vi "Main_v2_AE.vi"() -> ()   [LabVIEW 2023]
uses:
  AD2_MSO_SDK_class/MSOConfig.ctl
  AD2_MSO_SDK_class/AD2TriggerSources.ctl
  AD2_MSO_SDK_class/MSORangeCh.ctl
  AD2_DO_SDK_class/DOConfigureCustomData.ctl
  AD2_DO_SDK_class/DOTrigger.ctl
  AD2_WFG_SDK_class/AD2TriggerSources.ctl
  AD2_DO_SDK_class/DOCustomData.ctl
  Application_class/Application.lvclass
  <vilib>/Utility/error.llb/Error Cluster From Error Code.vi
  <vilib>/ErrorRing/Error Ring.xnode
  AD2_SDK_class/AD2_SDK.lvclass
  TC0608_class/TC0608.lvclass
  CetoniPump_class/CetoniPump.lvclass
  AFG3022B_class/AFG3022B.lvclass
  TBS2000Series_class/TBS2000Series.lvclass
  SaveData_class/SaveData.lvclass
  AD2_DO_SDK_class/AD2_DO_SDK.lvclass
  AD2_MSO_SDK_class/AD2_MSO_SDK.lvclass
panel:
  out "Pump Status":T1(array[cluster])
  in  "Tab Control":T2(tab)=enum."Log"
  out "Peltier is On":bool
  out "Oscilloscope is On":bool
  out "Analog Discovery (Camera Trigger) is On":bool
  out "Pump is On":bool
  out "Func is On":bool
  in  "Peltier Controller":bool
  in  "Oscilloscope":bool
  in  "Function Generator":bool
  in  "Cetoni Pump":bool
  in  "Analog Discovery":bool
  in  "Initialize Instruments":bool
  in  "Function Generator":refnum<visa-resource-name>
  in  "Oscilloscope":refnum<visa-resource-name>
  in  "Peltier VISA resource name":refnum<visa-resource-name>
  in  "Device Configuration Folder":string="C:\\Users\\Public\\Documents\\QmixElements\\Projects\\default_project\\Configurations\\sinle"
  in  "Oscilloscope Test":cluster{"Source Main":i32, "Source Probe":i32}={"Source Main"=2, "Source Probe"=1} {"Source Probe" items=["Math", "Channel 1", "Channel 2", "Channel 3", "Channel 4"]; "Source Main" items=["Math", "Channel 1", "Channel 2", "Channel 3", "Channel 4"]}
  in  "ReadOscilloscopeChannel":bool
  out "Temperature (C)":dbl
  in  "Read Peltier":bool
  in  "Frequency (1000 Hz)":dbl=1000.0
  in  "Set Frequency":bool
  in  "Voltage (1 Vpp)":dbl=1.0
  in  "Set Voltage":bool
  in  "Image  Aquisition":T3={"Minimum Time between frames(s)"=10.0, "Number of Frames"=0} {"Minimum Time between frames(s)" min=0.005}
  in  "Take Images":bool
  in  "Pump: GoToLevel":bool
  in  "GoToLevelSettings":T4
  in  "index":i32
  in  "refill below level":dbl
  in  "Timeout Refill":dbl=20.0 caption="Time Target (s)"
  in  "Pump: CheckLevel&Refill":bool
  in  "Pump: Reference Move":bool
  in  "Pump: Refill":bool
  in  "Index":i32
  in  "Pump: Empty":bool
  in  "Pump: Read Status":bool
  in  "SyringeSettings":T5={"Maximum Piston Stroke (mm)"=100.0, "Inner Diameter (mm)"=12.0}
  in  "index configure syringe":i32
  in  "Pump: Configure":bool
  in  "Pump: STOP":bool
  in  "Source (1: Channel 1)":i32(ring)=1 items=["Math", "Channel 1", "Channel 2", "Channel 3", "Channel 4"]
  out "Peak-to-Peak":dbl format="%.2p"
  out "Frequency":dbl format="%.2p"
  in  "MeasurePowerOsc":bool
  out "Oscilloscope Results Test":T6 {"Probe Current" format="%.2p"; "Phase Angle" format="%.2p"; "Main Freq" format="%.2p"; "Main Volt" format="%.2p"}
  in  "Oscilloscope":T7={"Source Main"=2, "Source Probe"=1, "Source Prefocus"=2} {"Source Prefocus" items=["Math", "Channel 1", "Channel 2", "Channel 3", "Channel 4"]; "Source Probe" items=["Math", "Channel 1", "Channel 2", "Channel 3", "Channel 4"]; "Source Main" items=["Math", "Channel 1", "Channel 2", "Channel 3", "Channel 4"]}
  in  "Start Experiment":bool
  out "Temperatur (C)":dbl
  in  "Experiment Settings":T8={"Frequencies (MHz)"=[], "Camera Settings"={"Minimum Time between\n frames(s)"=10.0, "Number of Frames"=0}, "Flowrates (ul/min)"=[], "Voltages (V)"=[]} {"Camera Settings"."Minimum Time between\n frames(s)" min=0.005}
  in  "SaveFolder":path
  out "Oscilloscope Results":T9 {"Probe Current" format="%.2p"; "Phase Angle" format="%.2p"; "Main Freq" format="%.2p"; "Main Volt" format="%.2p"; "Prefocus Freq" format="%.2p"; "Prefocus Volt" format="%.2p"}
  out "LOG":string
  in  "Change Frequencies and Measure":bool
  in  "FreqAndOscilloscopeTest":T10
  in  "Oscilloscope Source":i32(ring)=1 items=["Math", "Channel 1", "Channel 2", "Channel 3", "Channel 4"]
  out "Frequency (Osc.)":dbl format="%.2p"
  out "Voltage (Osc.)":dbl format="%.2p"
  out "Voltages":dbl
  out "Frequencies":dbl
  out "temperature (C)":dbl
  in  "Time To wait":dbl
  in  "Wait":bool
  in  "Configure MSO":bool
  in  "MSO":T11={"Timing"={"Enable"=TRUE, "Samples In"=100000.0, "Sample Rate"=1250000.0, "Mode"=enum."Single Sample"}, "Trigger"={"Hysteresis"=0.0, "Trigger Level"=0.0, "Trigger Condition"=0, "Trigger Type"=0, "Trigger Channel"=0, "secTimeout"=1.0, "TrigrSrc"=enum."trigrsrcNone"}, "Range Ch1"={"idxChannel"=0, "voltOffset"=0.0, "VoltsRange"=50}, "Range Ch 2"={"idxChannel"=1, "voltOffset"=0.0, "VoltsRange"=50}} {"Range Ch 2"."VoltsRange" items=["High 50V"=50, "Low5V"=5]; "Range Ch1"."VoltsRange" items=["High 50V"=50, "Low5V"=5]; "Trigger"."Trigger Channel" items=["Channel 1"=0, "Channel 2"=1, "Both"=-1]; "Trigger"."Trigger Type" items=["Edge", "Pulse", "Transition"]; "Trigger"."Trigger Condition" items=["Rising", "Falling"]}
  in  "Read MSO":bool
  out "Waveform Graph":waveform(dbl)[](graph)
  in  "Trigg AD2":bool
  in  "Configure DO":bool
  in  "?":T14={"DO Trigger"={"secRun(0=Cont)"=0.0, "secWait"=0.0, "cRepeat(0=inf)"=0, "Repeat Trigger"=TRUE, "TrigrSrc"=enum."trigsrcPC"}, "CustomData"=[{"Data"=[FALSE, TRUE, FALSE, FALSE, FALSE, FALSE, FALSE, FALSE, FALSE, FALSE, FALSE, FALSE, FALSE, FALSE, FALSE, FALSE, FALSE, FALSE, FALSE, FALSE, FALSE, FALSE], "Freq"=1000.0, "#Bits"=100, "Enable"=TRUE, "IdleState"=0}, {"Data"=[], "Freq"=0.0, "#Bits"=0, "Enable"=FALSE, "IdleState"=0}, {"Data"=[], "Freq"=0.0, "#Bits"=0, "Enable"=FALSE, "IdleState"=0}, {"Data"=[], "Freq"=0.0, "#Bits"=0, "Enable"=FALSE, "IdleState"=0}, {"Data"=[], "Freq"=0.0, "#Bits"=0, "Enable"=FALSE, "IdleState"=0}, {"Data"=[], "Freq"=0.0, "#Bits"=0, "Enable"=FALSE, "IdleState"=0}, {"Data"=[], "Freq"=0.0, "#Bits"=0, "Enable"=FALSE, "IdleState"=0}, {"Data"=[], "Freq"=0.0, "#Bits"=0, "Enable"=FALSE, "IdleState"=0}, {"Data"=[], "Freq"=0.0, "#Bits"=0, "Enable"=FALSE, "IdleState"=0}, {"Data"=[], "Freq"=0.0, "#Bits"=0, "Enable"=FALSE, "IdleState"=0}, {"Data"=[], "Freq"=0.0, "#Bits"=0, "Enable"=FALSE, "IdleState"=0}, {"Data"=[], "Freq"=0.0, "#Bits"=0, "Enable"=FALSE, "IdleState"=0}, {"Data"=[], "Freq"=0.0, "#Bits"=0, "Enable"=FALSE, "IdleState"=0}, {"Data"=[FALSE, FALSE, FALSE, FALSE, FALSE, FALSE, FALSE, FALSE, FALSE, FALSE, FALSE, FALSE, FALSE, FALSE, FALSE, FALSE, FALSE, FALSE, FALSE, FALSE, FALSE, FALSE, FALSE], "Freq"=0.0, "#Bits"=0, "Enable"=FALSE, "IdleState"=0}, {"Data"=[FALSE, FALSE, FALSE, FALSE, FALSE, FALSE, FALSE, FALSE, FALSE, FALSE, FALSE, FALSE, FALSE, FALSE, FALSE, FALSE, FALSE, FALSE, FALSE, FALSE, FALSE, FALSE, FALSE], "Freq"=0.0, "#Bits"=0, "Enable"=FALSE, "IdleState"=0}]}
  in  "ABORT":bool
  out "Status":string="Program Started\nPlease connect to instruments"
  out "error out":errorcluster
  in  "Exit":bool
  # "Notes: \nChange frequency input to MHz\ninvestigate index in GoToLevelSettings, might be unneccesary"
  # "Instruments"
  # "Peltier"
  # "Camera"
  # "Pump"
  # "Function Generator"
  # "Oscilloscope"
  # "Not sure if this is needed if we read the oscilloscope manually instead"
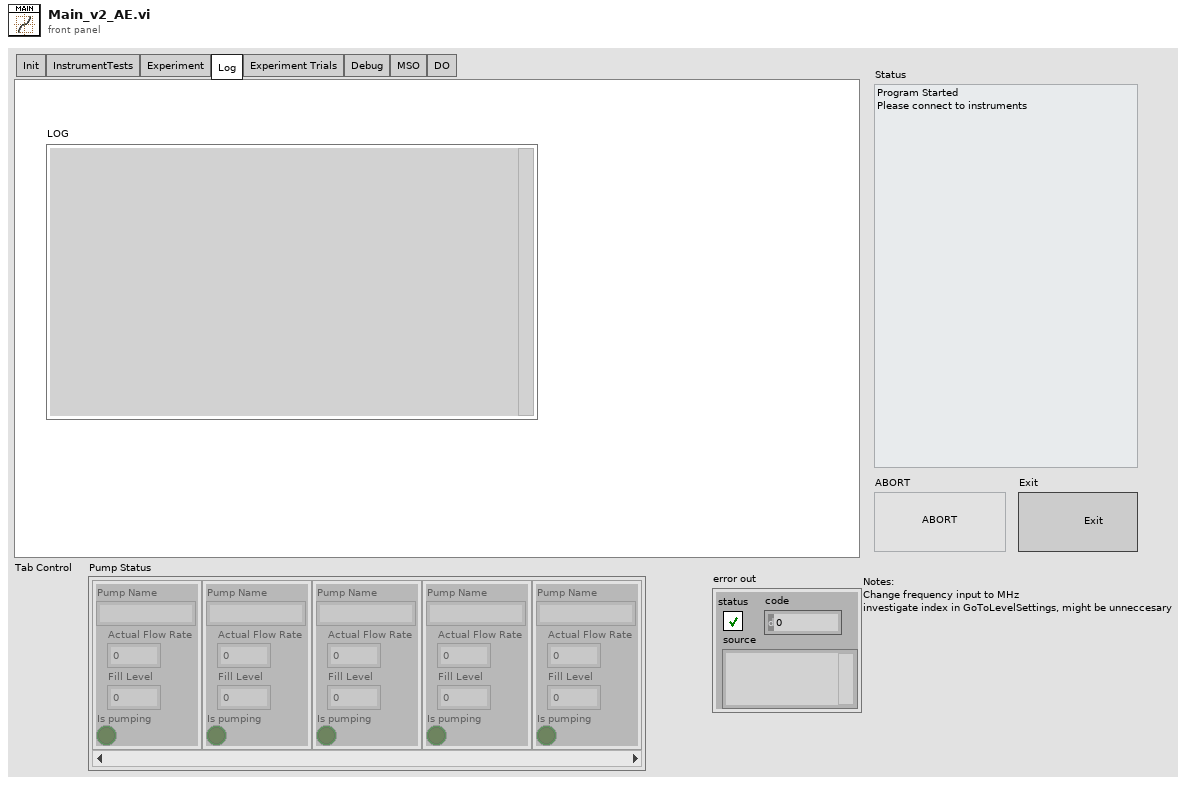
[diagram p1: front panel]
types:
  T1 = cluster{"Pump Name":string, "Actual Flow Rate":dbl, "Fill Level":dbl, "Is pumping":bool}[]
  T2 = enum32{"Init", "InstrumentTests", "Experiment", "Log", "Experiment Trials", "Debug", "MSO", "DO"}
  T3 = cluster{"Minimum Time between frames(s)":dbl, "Number of Frames":i32}
  T4 = cluster{"index":i32, "Level(ml)":dbl, "Flow":dbl}
  T5 = cluster{"Maximum Piston Stroke (mm)":dbl, "Inner Diameter (mm)":dbl}
  T6 = cluster{"Main Volt":dbl, "Main Freq":dbl, "Phase Angle":dbl, "Probe Current":dbl, "Power (Watt)":dbl}
  T7 = cluster{"Source Main":i32, "Source Probe":i32, "Source Prefocus":i32}
  T8 = cluster{"Frequencies (MHz)":dbl[], "Camera Settings":cluster{"Minimum Time between\n frames(s)":dbl, "Number of Frames":i32}, "Flowrates (ul/min)":dbl[], "Voltages (V)":dbl[]}
  T9 = cluster{"Prefocus":cluster{"Initial X":dbl, "X Increment":dbl, "Waveform Array":dbl[]}, "Prefocus Volt":dbl, "Prefocus Freq":dbl, "Main":cluster{"Initial X":dbl, "X Increment":dbl, "Waveform Array":dbl[]}, "Main Volt":dbl, "Main Freq":dbl, "Phase Angle":dbl, "Probe Current":dbl, "Power (Watt)":dbl}
  T10 = cluster{"Frequencies (MHz)":dbl[], "Voltages (V)":dbl[]}
  T11 = typedef "AD2_MSO_SDK.lvclass/MSOConfig.ctl" = cluster{"Timing":cluster{"Enable":bool, "Samples In":dbl, "Sample Rate":dbl, "Mode":enum16{"Single Sample", "Scanshift", "Multiple Samples", "Scan Screen"}}, "Trigger":cluster{"Hysteresis":dbl, "Trigger Level":dbl, "Trigger Condition":i32, "Trigger Type":i32, "Trigger Channel":i32, "secTimeout":dbl, "TrigrSrc":T12}, "Range Ch1":T13, "Range Ch 2":T13}
  T12 = typedef "AD2_MSO_SDK.lvclass/AD2TriggerSources.ctl" = enum8{"trigrsrcNone", "trigsrcPC", "trigsrcDetectorAnalogIn", "trigsrcDetectorDigitalIn", "trigsrcAnalogIn", "trigsrcDigitalIn", "trigsrcDigitalOut", "trigsrcAnalogOut1", "trigsrcAnalogOut2", "trigsrcAnalogOut3", "trigsrcAnalogOut4", "trigsrcExternal1", "trigsrcExternal2", "trigsrcExternal3", "trigsrcExternal4", ""}
  T13 = typedef "AD2_MSO_SDK.lvclass/MSORangeCh.ctl" = cluster{"idxChannel":i32, "voltOffset":dbl, "VoltsRange":u16}
  T14 = typedef "DOConfigureCustomData.ctl" = cluster{"DO Trigger":T15, "CustomData":T17}
  T15 = typedef "AD2_DO_SDK.lvclass/DOTrigger.ctl" = cluster{"secRun(0=Cont)":dbl, "secWait":dbl, "cRepeat(0=inf)":i32, "Repeat Trigger":bool, "TrigrSrc":T16}
  T16 = typedef "AD2_SDK.lvclass/AD2TriggerSources.ctl" = enum8{"trigrsrcNone", "trigsrcPC", "trigsrcDetectorAnalogIn", "trigsrcDetectorDigitalIn", "trigsrcAnalogIn", "trigsrcDigitalIn", "trigsrcDigitalOut", "trigsrcAnalogOut1", "trigsrcAnalogOut2", "trigsrcAnalogOut3", "trigsrcAnalogOut4", "trigsrcExternal1", "trigsrcExternal2", "trigsrcExternal3", "trigsrcExternal4", ""}
  T17 = typedef "AD2_DO_SDK.lvclass/DOCustomData.ctl" = cluster{"Data":bool[], "Freq":dbl, "#Bits":u32, "Enable":bool, "IdleState":u16}[]
  T18 = cluster{"Voltages":dbl, "Numeric":dbl, "selected path":path}
  T19 = cluster{"Minimum Time between frames":dbl, "Number of Frames":i32}
  T20 = cluster{"Pump Handle":i64, "Pump Name":string, "Maximum Volume":dbl, "Maximum Flow Rate":dbl, "Flow Rate":dbl, "Target Level":dbl, "Valve Handle":i64, "Has Valve?":bool, "Actual valve position":i32}[]
  T21 = cluster{"Frequency":dbl, "Peak-to-Peak":dbl, "temperature (C)":dbl}
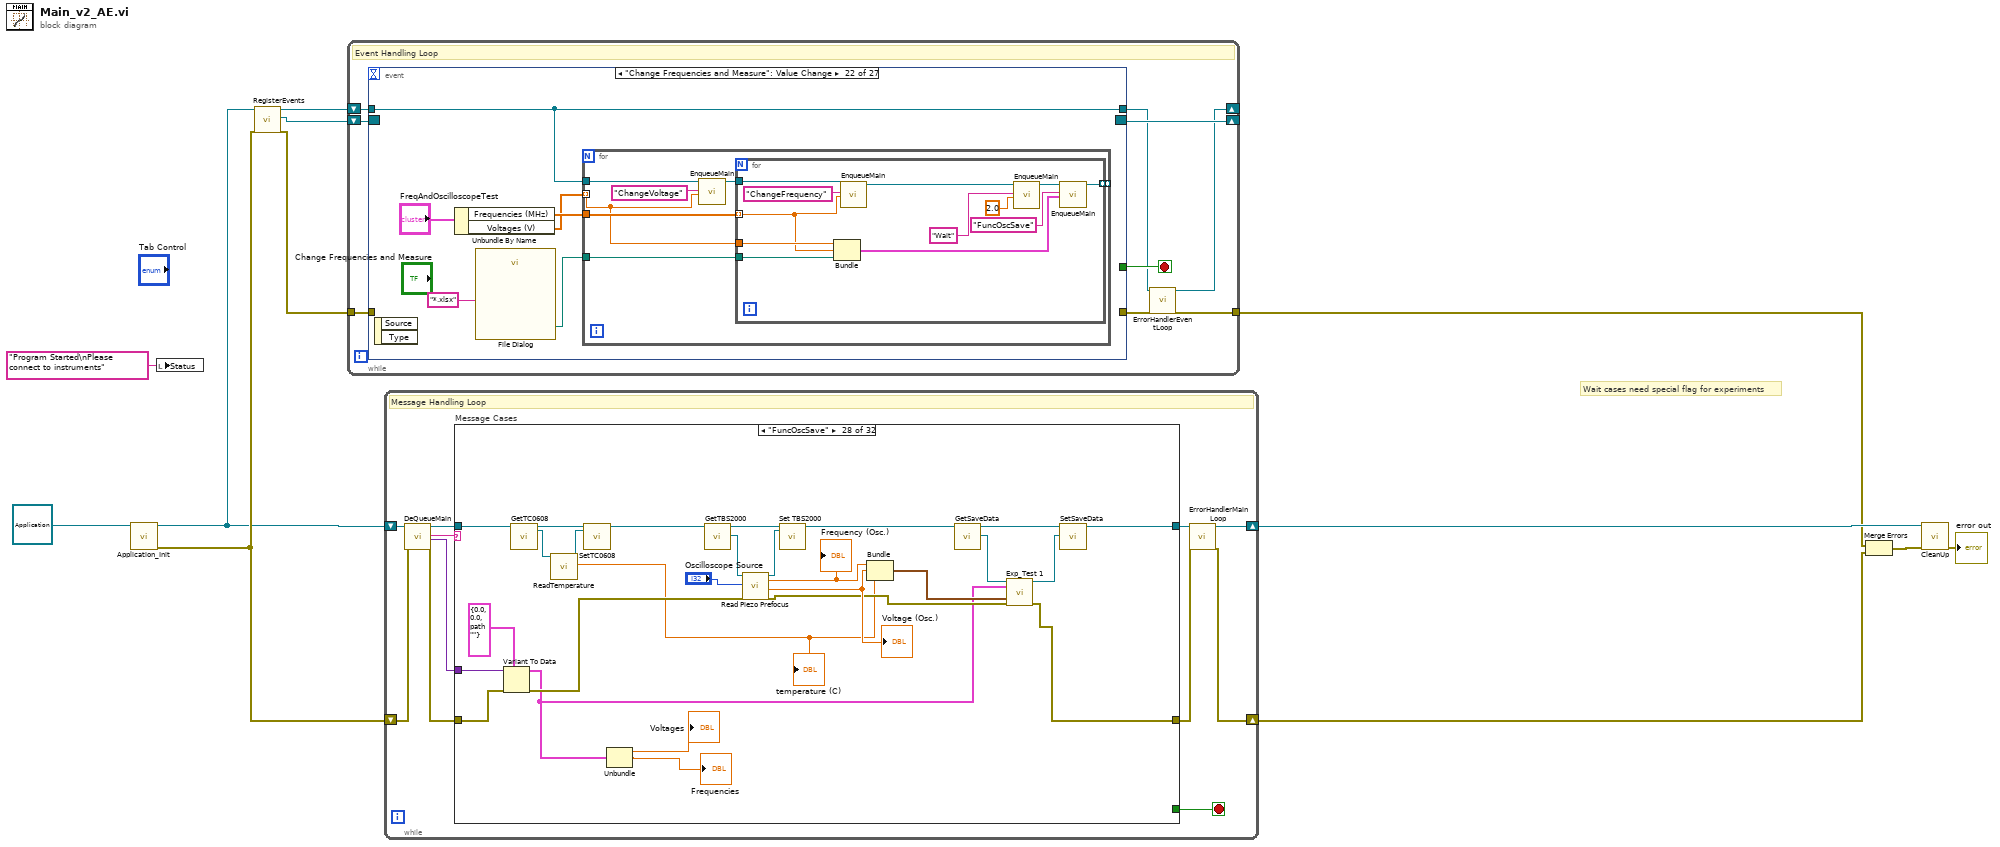
[diagram p0: block diagram]
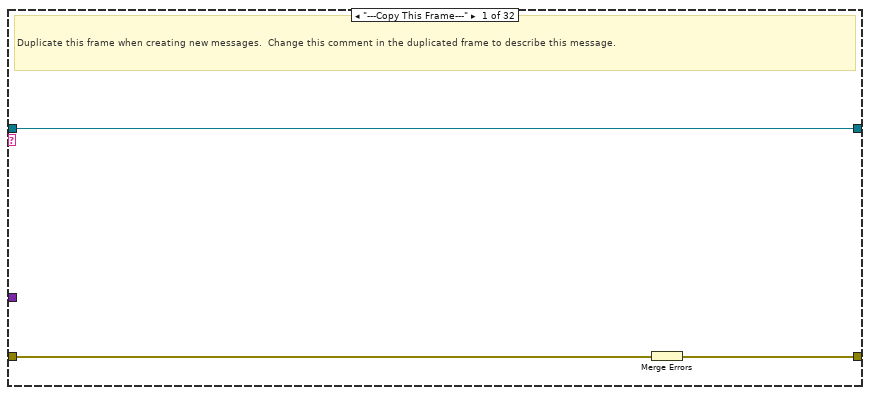
[diagram p2: hidden frame]
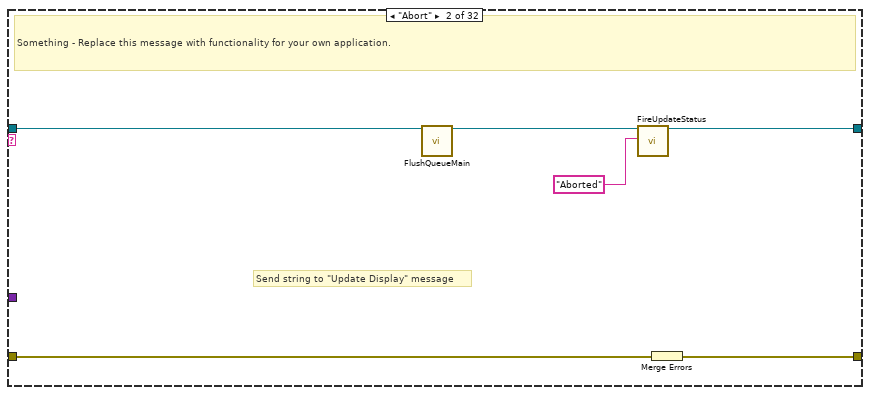
[diagram p3: hidden frame]
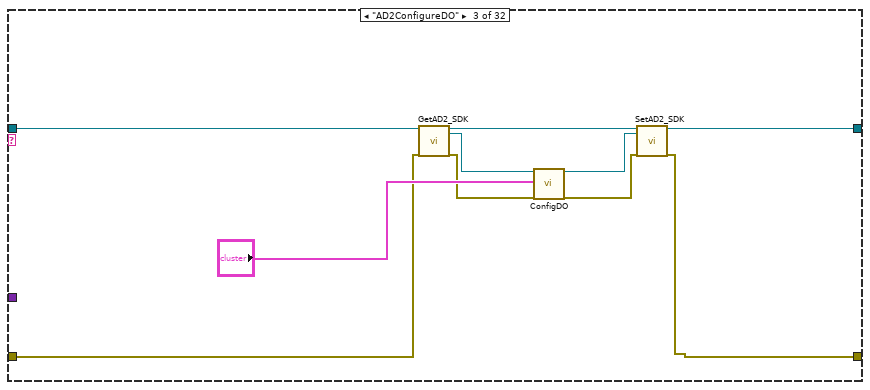
[diagram p4: hidden frame]
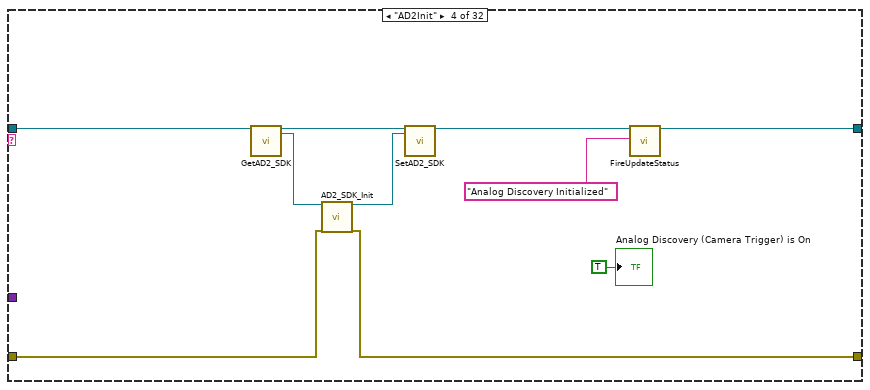
[diagram p5: hidden frame]
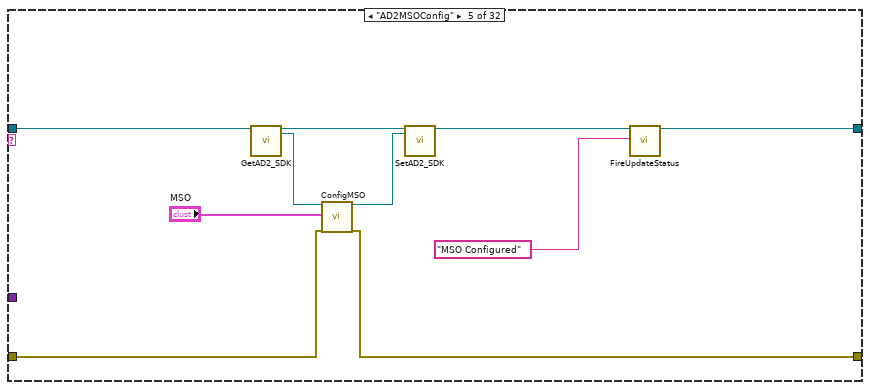
[diagram p6: hidden frame]
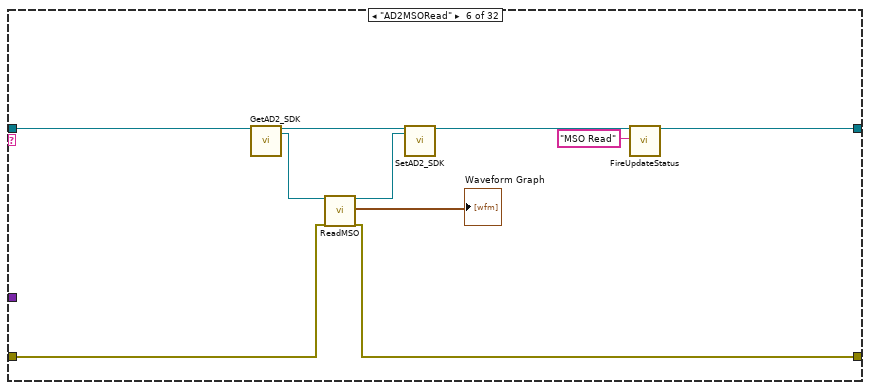
[diagram p7: hidden frame]
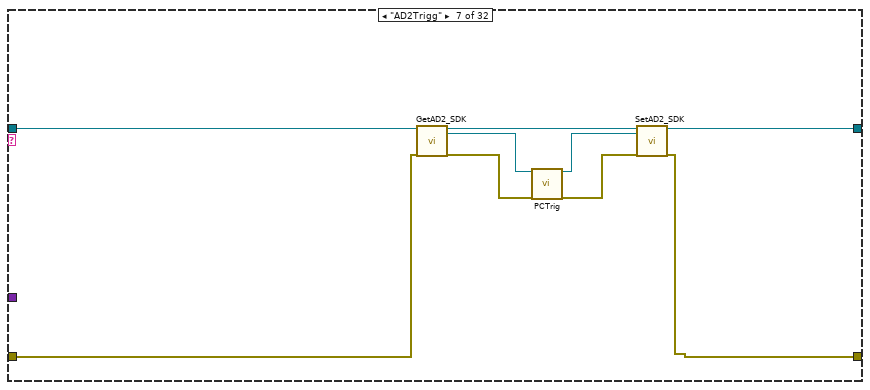
[diagram p8: hidden frame]
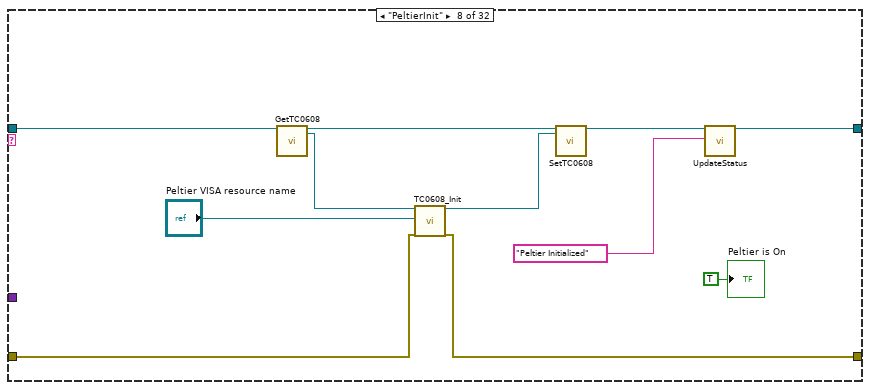
[diagram p9: hidden frame]
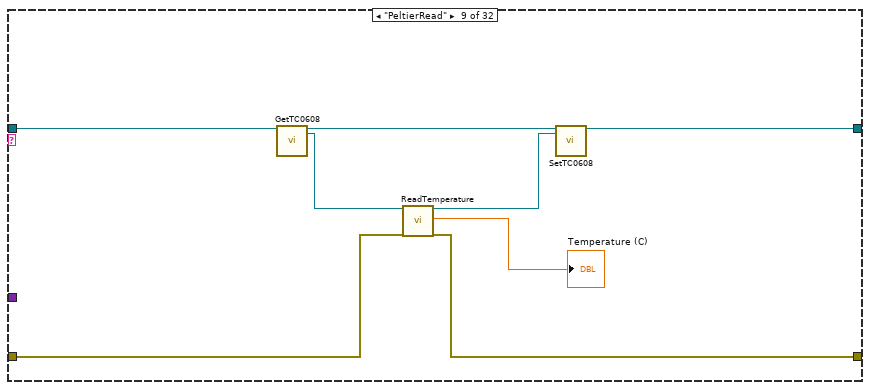
[diagram p10: hidden frame]
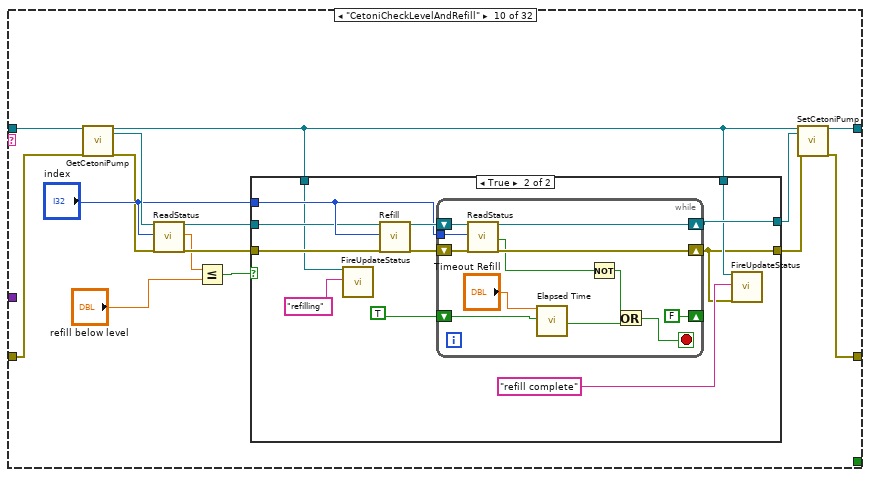
[diagram p11: hidden frame]
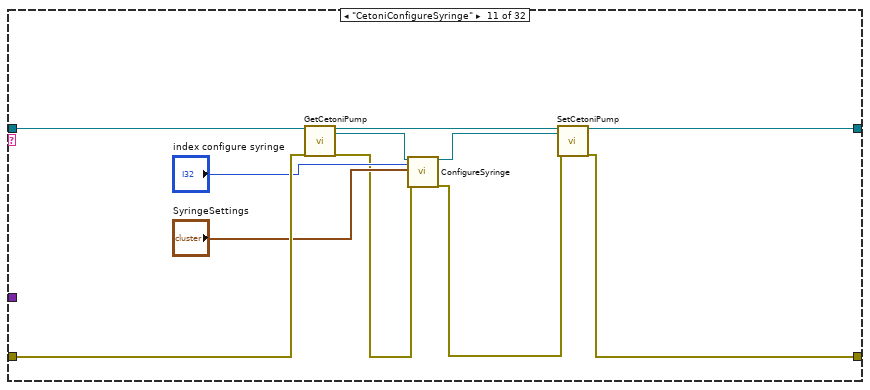
[diagram p13: hidden frame]
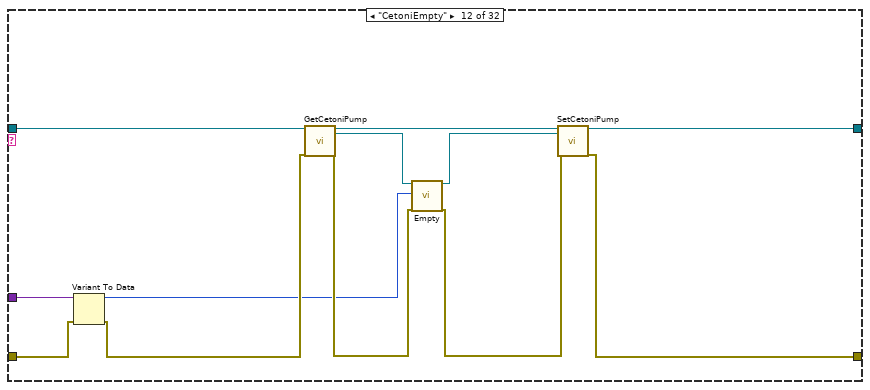
[diagram p14: hidden frame]
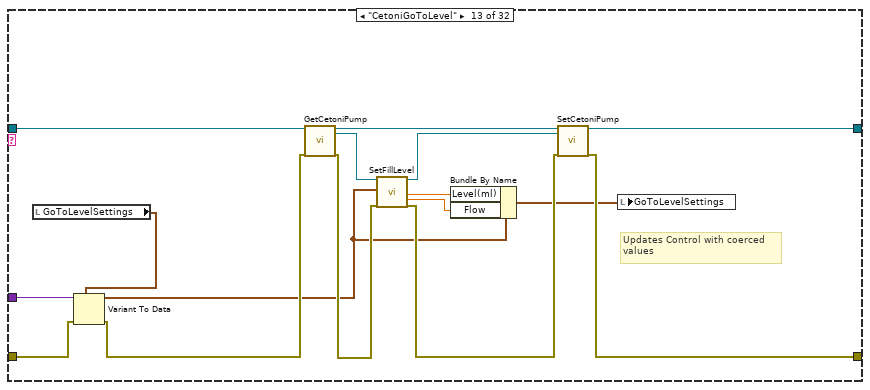
[diagram p15: hidden frame]
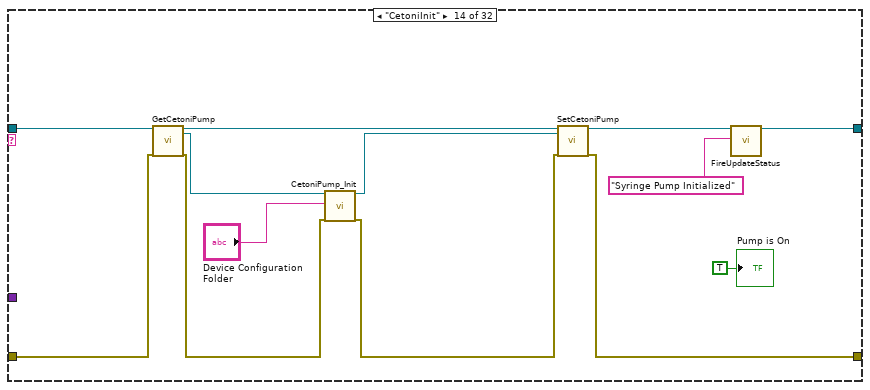
[diagram p16: hidden frame]
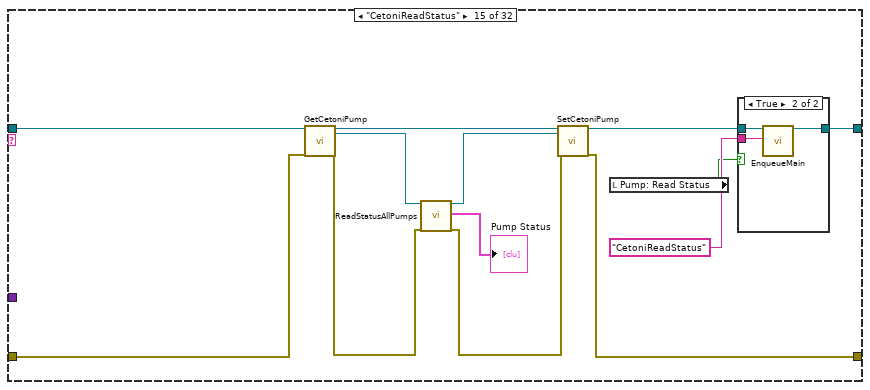
[diagram p17: hidden frame]
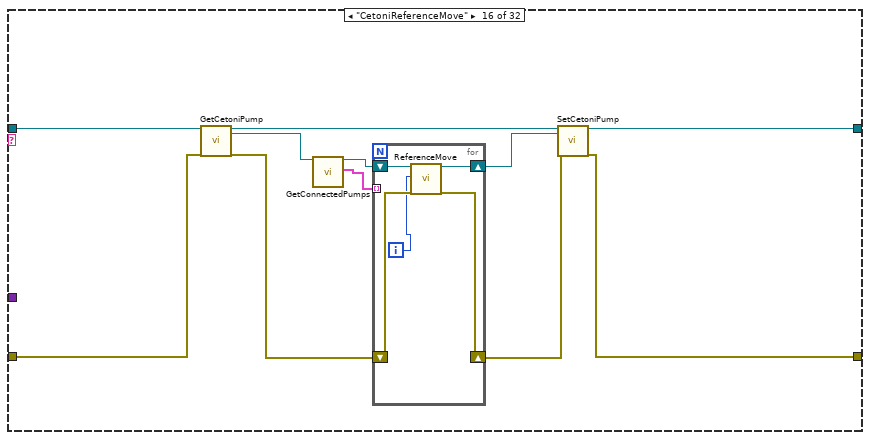
[diagram p19: hidden frame]
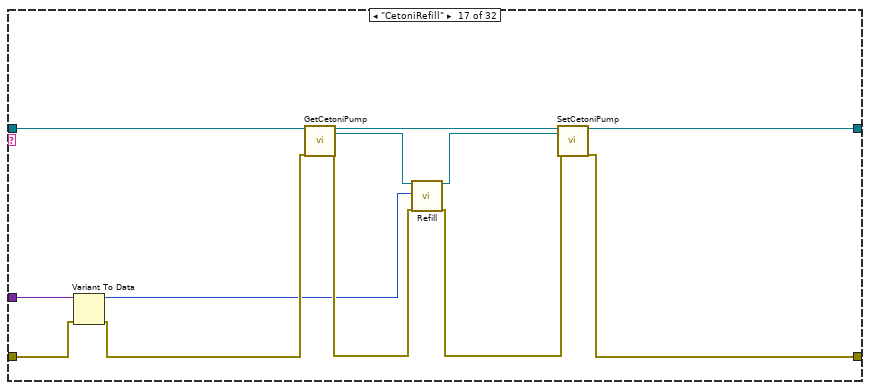
[diagram p20: hidden frame]
diagram:
  # "Wait cases need special flag for experiments"
  n1 = call "Application_Init.vi"("object in"=refnum<class "Application.lvclass"> refnum ("Application")) -> ("object out"=w2:refnum<class "Application.lvclass">, "error out"=w8:errorcluster)  [unwired: 17 in]
  n2 = local write "Status"("Program Started\nPlease connect to instruments" ("Status")) -> ()
  n3 = call-dynamic "RegisterEvents.vi"("object in"=w2, "error in (no error)"=w8) -> ("object out"=w10:refnum<class "Application.lvclass">, "Event Registration Refnum"=w11:refnum<event-registration>, "error out"=w9:errorcluster)  [unwired: 15 in]
  n4 = while {
    shift-right: [w20] -> _
    shift-left: w11 -> [w21]
    tunnel: [w15] -> w5
    shift-right: [w13] -> _
    shift-left: w10 -> [w18]
    tunnel: w9 -> [w17]
    stop <- w19 stop-if-true
    # "Event Handling Loop"
    n5 = event shown="[21] \"Change Frequencies and Measure\": Value Change" {
      selector: w21 -> [_ _ _ _ _ _ _ _ _ _ _ _ _ _ _ _ _ _ _ _ _ _ _ _ _ _ _]
      dyn-events: [_ _ _ _ _ _ _ _ _ _ _ _ _ _ _ _ _ _ _ _ _ _ _ _ _ _ _] -> w20
      timeout: _ -> [_ _ _ _ _ _ _ _ _ _ _ _ _ _ _ _ _ _ _ _ _ _ _ _ _ _ _]
      tunnel: [TRUE ("Discard?") _ _ _ _ _ _ _ _ _ _ _ _ _ _ _ _ _ _ _ _ _ _ _ _ _ _] -> w19
      tunnel: [w23 w29 w37 w42 _ _ w84 _ _ _ _ _ w104 w110 w116 w122 w127 w134 _ _ _ _ _ _ _ _ w191] -> w16
      tunnel: w18 -> [w28 w34 w36 w43 w47 w49 w88 w91 w94 w96 w98 w102 w105 w111 w117 w123 w128 w135 w146 w149 w151 w155 w180 w183 w186 w189 w194]
      tunnel: [w27 w33 w35 w43 w46 w50 w87 w91 w94 w96 w98 w101 w106 w112 w118 w124 w129 w136 w145 w148 w152 w155 w179 w182 w185 w188 w194] -> w14
      tunnel: w17 -> [w24 w30 w38 w42 _ _ w85 _ _ _ _ _ w103 w109 w115 w121 w126 w133 _ _ _ _ _ _ _ _ w192]
      event "Exit": Value Change {
        (unwired) "\"Exit\" button pressed" ("VI Stopped")
        n6 = event-data() -> ()  [unwired: 1 in, 1 out]
        n7 = call-dynamic "EnqueueMain.vi"("object in"=w28, "Message"="Exit", "error in (no error)"=w24, "Priority Message? (F)"=TRUE) -> ("object out"=w27:refnum<class "Application.lvclass">, "error out"=w23:errorcluster)  [unwired: 14 in]
      }
      event "ABORT": Value Change {
        n8 = event-data() -> ()  [unwired: 1 in, 1 out]
        n9 = call-dynamic "EnqueueMain.vi"("object in"=w34, "Message"="Abort", "error in (no error)"=w30, "Priority Message? (F)"=TRUE) -> ("object out"=w33:refnum<class "Application.lvclass">, "error out"=w29:errorcluster)  [unwired: 14 in]
      }
      event Panel Close? {
        # "Send the 'Confirm Quit' message if the user closes the panel of the VI. Discard the event so the 'Confirm Quit' message has a chance to run."
        n10 = event-data() -> ()  [unwired: 1 in, 1 out]
        n11 = call-dynamic "EnqueueMain.vi"("object in"=w36, "Message"="Confirm Quit", "error in (no error)"=w38, "Priority Message? (F)"=TRUE) -> ("object out"=w35:refnum<class "Application.lvclass">, "error out"=w37:errorcluster)  [unwired: 14 in]
        n12 = event-data("Discard?"=TRUE) -> ()  [unwired: 1 in, 1 out]
      }
      event Application Instance Close {
        # "stop the pumps if it's not automatically build into the cetoni software\nsave the log to a file"
        # "#CodeRecommended - When a project closes, all VIs within that project are aborted and leave memory. However, any code placed in this event frame is guaranteed to run to completion, so add any cleanup code that absolutely must happen here."
        n13 = event-data() -> ()  [unwired: 1 in, 1 out]
      }
      event "Wait": Value Change {
        n14 = event-data() -> ()  [unwired: 1 in, 2 out]
        n15 = call-dynamic "EnqueueMain.vi"("object in"=w47, "Message"="Wait", "Message Data"="Time To wait") -> ("object out"=w46:refnum<class "Application.lvclass">)  [unwired: 15 in, 1 out]
      }
      event "Initialize Instruments": Value Change {
        n16 = event-data() -> ()  [unwired: 1 in, 2 out]
        n17 = case shown="False" "Function Generator" {
          tunnel: w49 -> [w80 w83]
          tunnel: [w80 w82] -> w63
          tunnel: "FuncInit" ("Message") -> [_ w81]
          frame False {
          }
          frame True {
            n18 = call-dynamic "EnqueueMain.vi"("object in"=w83, "Message"=w81) -> ("object out"=w82:refnum<class "Application.lvclass">)  [unwired: 16 in, 1 out]
          }
        }
        n19 = case shown="False" "Cetoni Pump" {
          tunnel: w63 -> [w76 w79]
          tunnel: "CetoniInit" ("Message") -> [_ w78]
          tunnel: [w76 w77] -> w60
          frame False {
          }
          frame True {
            n20 = call-dynamic "EnqueueMain.vi"("object in"=w79, "Message"=w78) -> ("object out"=w77:refnum<class "Application.lvclass">)  [unwired: 16 in, 1 out]
          }
        }
        n21 = case shown="True" "Analog Discovery" {
          tunnel: w60 -> [w72 w75]
          tunnel: "AD2Init" ("Message") -> [_ w74]
          tunnel: [w72 w73] -> w56
          frame False {
          }
          frame True {
            n22 = call-dynamic "EnqueueMain.vi"("object in"=w75, "Message"=w74) -> ("object out"=w73:refnum<class "Application.lvclass">)  [unwired: 16 in, 1 out]
          }
        }
        n23 = case shown="True" "Oscilloscope" {
          tunnel: w56 -> [w68 w71]
          tunnel: "OscilloscopeInit" ("Message") -> [_ w70]
          tunnel: [w68 w69] -> w53
          frame False {
          }
          frame True {
            n24 = call-dynamic "EnqueueMain.vi"("object in"=w71, "Message"=w70) -> ("object out"=w69:refnum<class "Application.lvclass">)  [unwired: 16 in, 1 out]
          }
        }
        n25 = case shown="True" "Peltier Controller" {
          tunnel: w53 -> [w64 w67]
          tunnel: "PeltierInit" ("Message") -> [_ w66]
          tunnel: [w64 w65] -> w50
          frame False {
          }
          frame True {
            n26 = call-dynamic "EnqueueMain.vi"("object in"=w67, "Message"=w66) -> ("object out"=w65:refnum<class "Application.lvclass">)  [unwired: 16 in, 1 out]
          }
        }
      }
      event "Read Peltier": Value Change {
        n27 = event-data() -> ()  [unwired: 1 in, 2 out]
        n28 = call-dynamic "EnqueueMain.vi"("object in"=w88, "Message"="PeltierRead", "error in (no error)"=w85) -> ("object out"=w87:refnum<class "Application.lvclass">, "error out"=w84:errorcluster)  [unwired: 15 in]
      }
      event "Set Frequency": Value Change {
        n29 = event-data() -> ()  [unwired: 1 in, 2 out]
        n30 = call-dynamic "EnqueueMain.vi"("object in"=w91, "Message"="ChangeFrequency", "Message Data"="Frequency (1000 Hz)") -> ()  [unwired: 15 in, 2 out]
      }
      event "Set Voltage": Value Change {
        n31 = event-data() -> ()  [unwired: 1 in, 2 out]
        n32 = call-dynamic "EnqueueMain.vi"("object in"=w94, "Message"="ChangeVoltage", "Message Data"="Voltage (1 Vpp)") -> ()  [unwired: 15 in, 2 out]
      }
      event "MeasurePowerOsc": Value Change {
        n33 = event-data() -> ()  [unwired: 1 in, 2 out]
        n34 = call-dynamic "EnqueueMain.vi"("object in"=w96, "Message"="MeasurePowerOsc") -> ()  [unwired: 16 in, 2 out]
      }
      event "ReadOscilloscopeChannel": Value Change {
        n35 = event-data() -> ()  [unwired: 1 in, 2 out]
        n36 = call-dynamic "EnqueueMain.vi"("object in"=w98, "Message"="ReadOscilloscopeChannel") -> ()  [unwired: 16 in, 2 out]
      }
      event "Take Images": Value Change {
        n37 = event-data() -> ()  [unwired: 1 in, 2 out]
        n38 = call-dynamic "EnqueueMain.vi"("object in"=w102, "Message"="TakeNImages", "Message Data"="Image  Aquisition") -> ("object out"=w101:refnum<class "Application.lvclass">)  [unwired: 15 in, 1 out]
      }
      event "Pump: Configure": Value Change {
        n39 = event-data() -> ()  [unwired: 1 in, 2 out]
        n40 = call-dynamic "EnqueueMain.vi"("object in"=w105, "Message"="CetoniConfigureSyringe", "error in (no error)"=w103) -> ("object out"=w106:refnum<class "Application.lvclass">, "error out"=w104:errorcluster)  [unwired: 15 in]
      }
      event "Pump: GoToLevel": Value Change {
        n41 = event-data() -> ()  [unwired: 1 in, 2 out]
        n42 = call-dynamic "EnqueueMain.vi"("object in"=w111, "Message"="CetoniGoToLevel", "Message Data"="GoToLevelSettings", "error in (no error)"=w109) -> ("object out"=w112:refnum<class "Application.lvclass">, "error out"=w110:errorcluster)  [unwired: 14 in]
      }
      event "Pump: Empty": Value Change {
        n43 = event-data() -> ()  [unwired: 1 in, 2 out]
        n44 = local read "Index"() -> (w114:i32)
        n45 = call-dynamic "EnqueueMain.vi"("object in"=w117, "Message"="CetoniEmpty", "Message Data"=w114, "error in (no error)"=w115) -> ("object out"=w118:refnum<class "Application.lvclass">, "error out"=w116:errorcluster)  [unwired: 14 in]
      }
      event "Pump: Refill": Value Change {
        n46 = event-data() -> ()  [unwired: 1 in, 2 out]
        n47 = call-dynamic "EnqueueMain.vi"("object in"=w123, "Message"="CetoniRefill", "Message Data"="Index", "error in (no error)"=w121) -> ("object out"=w124:refnum<class "Application.lvclass">, "error out"=w122:errorcluster)  [unwired: 14 in]
      }
      event "Pump: Read Status": Value Change {
        n48 = event-data() -> ()  [unwired: 1 in, 2 out]
        n49 = call-dynamic "EnqueueMain.vi"("object in"=w128, "Message"="CetoniReadStatus", "error in (no error)"=w126) -> ("object out"=w129:refnum<class "Application.lvclass">, "error out"=w127:errorcluster)  [unwired: 15 in]
      }
      event "Pump: Reference Move": Value Change {
        n50 = event-data() -> ()  [unwired: 1 in, 2 out]
        n51 = Two Button Dialog(message="The pumps will perform a reference move. Please remove all syringes!!!!! ") -> (T button?=w132:bool)  [unwired: 2 in]
        n52 = case shown="True" w132 {
          tunnel: [w137 w142] -> w136
          tunnel: w135 -> [w137 w141]
          tunnel: [w138 w140] -> w134
          tunnel: w133 -> [w138 w139]
          frame False {
          }
          frame True {
            n53 = call-dynamic "EnqueueMain.vi"("object in"=w141, "Message"="CetoniReferenceMove", "error in (no error)"=w139) -> ("object out"=w142:refnum<class "Application.lvclass">, "error out"=w140:errorcluster)  [unwired: 15 in]
          }
        }
      }
      event "Pump: CheckLevel&Refill": Value Change {
        n54 = event-data() -> ()  [unwired: 1 in, 2 out]
        n55 = call-dynamic "EnqueueMain.vi"("object in"=w146, "Message"="CetoniCheckLevelAndRefill") -> ("object out"=w145:refnum<class "Application.lvclass">)  [unwired: 16 in, 1 out]
      }
      event "Pump: STOP": Value Change {
        n56 = event-data() -> ()  [unwired: 1 in, 2 out]
        n57 = call-dynamic "EnqueueMain.vi"("object in"=w149, "Message"="CetoniStopPumps") -> ("object out"=w148:refnum<class "Application.lvclass">)  [unwired: 16 in, 1 out]
      }
      event "Start Experiment": Value Change {
        # "I made a Subvi to fit screen"
        n58 = event-data() -> ()  [unwired: 1 in, 2 out]
        n59 = call-dynamic "BuildExperiment.vi"("object in"=w151, "Experiment Settings"="Experiment Settings") -> ("object out"=w152:refnum<class "Application.lvclass">)  [unwired: 16 in, 1 out]
      }
      event "Change Frequencies and Measure": Value Change {
        n60 = event-data() -> ()  [unwired: 1 in, 2 out]
        n61 = Unbundle By Name("FreqAndOscilloscopeTest") -> ("Frequencies (MHz)"=w157:dbl[], "Voltages (V)"=w156:dbl[])
        n62 = call "File Dialog"("pattern (all files)"="*.xlsx") -> ("selected path"=w153:path)  [unwired: 11 in, 3 out]
        n63 = for {
          tunnel: w157 -> [w165]
          tunnel: w156 -> [w164] mode=indexing
          tunnel: w155 -> [w163]
          tunnel: [w161] -> _ mode=indexing
          tunnel: w153 -> [w159]
          n64 = call-dynamic "EnqueueMain.vi"("object in"=w163, "Message"="ChangeVoltage", "Message Data"=w164) -> ("object out"=w162:refnum<class "Application.lvclass">)  [unwired: 15 in, 1 out]
          n65 = for {
            tunnel: w165 -> [w168] mode=indexing
            tunnel: w164 -> [w169]
            tunnel: w162 -> [w177]
            tunnel: [w176] -> w161 mode=indexing
            tunnel: w159 -> [w167]
            n66 = Bundle("Voltages"=w169, "Numeric"=w168, "selected path"=w167) -> (w166:T18)  [unwired: 1 in]
            n67 = call-dynamic "EnqueueMain.vi"("object in"=w177, "Message"="ChangeFrequency", "Message Data"=w168) -> ("object out"=w174:refnum<class "Application.lvclass">)  [unwired: 15 in, 1 out]
            n68 = call-dynamic "EnqueueMain.vi"("object in"=w174, "Message"="Wait", "Message Data"=2.0 ("Time to wait")) -> ("object out"=w173:refnum<class "Application.lvclass">)  [unwired: 15 in, 1 out]
            n69 = call-dynamic "EnqueueMain.vi"("object in"=w173, "Message"="FuncOscSave", "Message Data"=w166) -> ("object out"=w176:refnum<class "Application.lvclass">)  [unwired: 15 in, 1 out]
          }
        }
      }
      event "Configure DO": Value Change {
        n70 = event-data() -> ()  [unwired: 1 in, 2 out]
        n71 = call-dynamic "EnqueueMain.vi"("object in"=w180, "Message"="AD2ConfigureDO") -> ("object out"=w179:refnum<class "Application.lvclass">)  [unwired: 16 in, 1 out]
      }
      event "Configure MSO": Value Change {
        n72 = event-data() -> ()  [unwired: 1 in, 2 out]
        n73 = call-dynamic "EnqueueMain.vi"("object in"=w183, "Message"="AD2MSOConfig") -> ("object out"=w182:refnum<class "Application.lvclass">)  [unwired: 16 in, 1 out]
      }
      event "Read MSO": Value Change {
        n74 = event-data() -> ()  [unwired: 1 in, 2 out]
        n75 = call-dynamic "EnqueueMain.vi"("object in"=w186, "Message"="AD2MSORead") -> ("object out"=w185:refnum<class "Application.lvclass">)  [unwired: 16 in, 1 out]
      }
      event "Trigg AD2": Value Change {
        n76 = event-data() -> ()  [unwired: 1 in, 2 out]
        n77 = call-dynamic "EnqueueMain.vi"("object in"=w189, "Message"="AD2Trigg") -> ("object out"=w188:refnum<class "Application.lvclass">)  [unwired: 16 in, 1 out]
      }
      event User Event {
        n78 = event-data() -> ("Message"=w193:string, "Message Data"=w190:variant)  [unwired: 1 in]
        n79 = case shown="\"UpdateStatus\"" w193 {
          tunnel: w192 -> [w198 w207]
          tunnel: [w198 w207] -> w191
          tunnel: w190 -> [w197 _]
          frame "UpdateStatus" {
            # "I have disabled the log, it might slow down the program\nwhen it becomes to large"
            n80 = Variant To Data(type="" ("Status"), Variant=w197) -> (data=w195:string)  [unwired: 1 in, 1 out]
            "Status" <- w195
            n81 = disable-structure shown="Disabled" {
              disable-tunnel: w195 -> [w202 _]
              frame Disabled {
                n82 = Get Date/Time In Seconds() -> (seconds since 1Jan1904=w206:timestamp)
                n83 = Get Date/Time String(seconds (now)=w206) -> (time string=w203:string)  [unwired: 2 in, 1 out]
                n84 = feedback #1("" ("string")) -> (w199:string)
                n85 = Concatenate Strings(w199, "\r", w203, "\t", w202) -> (w201:string)
                "LOG" <- w201
                n86 = feedback-in #1(w201) -> ()
              }
              frame Enabled {
              }
            }
          }
          frame Default {
          }
        }
      }
    }
    n87 = call-dynamic "ErrorHandlerEventLoop.vi"("object in"=w14, "error in (no error)"=w16) -> ("object out"=w13:refnum<class "Application.lvclass">, "error out"=w15:errorcluster)  [unwired: 16 in]
  }
  n88 = while {
    shift-right: [w211] -> w7
    shift-left: w2 -> [w217]
    shift-right: [w212] -> w6
    shift-left: w8 -> [w208]
    stop <- w218 stop-if-true
    # "Message Handling Loop"
    n89 = call-dynamic "DeQueueMain.vi"("object in"=w217, "error in (no error)"=w208) -> ("object out"=w216:refnum<class "Application.lvclass">, "Message"=w215:string, "Message Data"=w214:variant, "error out"=w209:errorcluster)  [unwired: 14 in]
    n90 = case "Message Cases" shown="\"FuncOscSave\"" w215 {
      selector: w215 -> [_ _ _ _ _ _ _ _ _ _ _ _ _ _ _ _ _ _ _ _ _ _ _ _ _ _ _ _ _ _ _ w623]
      tunnel: w209 -> [w221 w226 w228 w243 w253 w262 w272 w280 w290 w307 w343 w353 w364 w387 w398 w412 w427 w438 w449 w465 w476 w478 w487 w503 w516 w519 w535 w551 w579 w587 w619 _]
      tunnel: [w220 w227 w229 w244 w254 w261 w273 w281 w289 w308 w345 w357 w373 w386 w400 w414 w431 w440 w450 w466 w471 w479 w488 w503 w515 w520 w535 w547 w568 w588 w615 w624] -> w213
      tunnel: [_ _ _ _ _ _ _ _ _ _ _ _ _ _ _ _ _ _ _ _ _ TRUE _ _ _ _ _ _ _ _ _ _] -> w218
      tunnel: w214 -> [_ _ _ _ _ _ _ _ _ _ _ w355 w366 _ _ _ w429 _ w451 w467 w475 _ _ _ _ _ _ w562 w566 w590 w621 _]
      tunnel: w216 -> [w219 w225 w237 w247 w257 w267 w276 w283 w293 w310 w347 w359 w375 w388 w401 w416 w433 w442 w452 w468 w470 w480 w492 w498 w513 w526 w532 w539 w583 w594 w617 w622]
      tunnel: [w219 w223 w235 w240 w249 w260 w274 w279 w294 w309 w346 w358 w374 w377 w390 w415 w432 w441 w447 w463 w470 w481 w484 w499 w509 w524 w533 w555 w571 w595 w612 w622] -> w210
      frame "---Copy This Frame---" {
        # "Duplicate this frame when creating new messages.  Change this comment in the duplicated frame to describe this message."
        n91 = Merge Errors(w221) -> (w220:errorcluster)
      }
      frame "Abort" {
        # "Send string to \"Update Display\" message"
        # "Something - Replace this message with functionality for your own application."
        n92 = call-dynamic "FlushQueueMain.vi"("object in"=w225) -> ("object out"=w224:refnum<class "Application.lvclass">)  [unwired: 16 in, 2 out]
        n93 = call-dynamic "FireUpdateStatus.vi"("object in"=w224, "Status"="Aborted") -> ("object out"=w223:refnum<class "Application.lvclass">)  [unwired: 16 in, 1 out]
        n94 = Merge Errors(w226) -> (w227:errorcluster)
      }
      frame "AD2ConfigureDO" {
        n95 = call-dynamic "GetAD2_SDK.vi"("object in"=w237, "error in (no error)"=w228) -> ("object out"=w236:refnum<class "Application.lvclass">, "AD2_SDK"=w233:refnum<class "AD2_SDK.lvclass">, "error out"=w232:errorcluster)  [unwired: 15 in]
        n96 = call-dynamic "ConfigDO.vi"("object in"=w233, 2:"?", "error in (no error)"=w232) -> ("object out"=w231:refnum<class "AD2_SDK.lvclass">, "error out"=w230:errorcluster)  [unwired: 15 in]
        n97 = call-dynamic "SetAD2_SDK.vi"("object in"=w236, "AD2_SDK"=w231, "error in (no error)"=w230) -> ("object out"=w235:refnum<class "Application.lvclass">, "error out"=w229:errorcluster)  [unwired: 15 in]
      }
      frame "AD2Init" {
        n98 = call-dynamic "GetAD2_SDK.vi"("object in"=w247) -> ("object out"=w246:refnum<class "Application.lvclass">, "AD2_SDK"=w242:refnum<class "AD2_SDK.lvclass">)  [unwired: 16 in, 1 out]
        n99 = call "AD2_SDK_Init.vi"("object in"=w242, "error in (no error)"=w243) -> ("object out"=w241:refnum<class "AD2_SDK.lvclass">, "error out"=w244:errorcluster)  [unwired: 16 in]
        n100 = call-dynamic "SetAD2_SDK.vi"("object in"=w246, "AD2_SDK"=w241) -> ("object out"=w245:refnum<class "Application.lvclass">)  [unwired: 16 in, 1 out]
        n101 = call-dynamic "FireUpdateStatus.vi"("object in"=w245, "Status"="Analog Discovery Initialized") -> ("object out"=w240:refnum<class "Application.lvclass">)  [unwired: 16 in, 1 out]
        "Analog Discovery (Camera Trigger) is On" <- TRUE ("Analog Discovery (Camera Trigger) is On")
      }
      frame "AD2MSOConfig" {
        n102 = call-dynamic "GetAD2_SDK.vi"("object in"=w257) -> ("object out"=w256:refnum<class "Application.lvclass">, "AD2_SDK"=w252:refnum<class "AD2_SDK.lvclass">)  [unwired: 16 in, 1 out]
        n103 = call-dynamic "ConfigMSO.vi"("object in"=w252, "variant"="MSO", "error in (no error)"=w253) -> ("object out"=w251:refnum<class "AD2_SDK.lvclass">, "error out"=w254:errorcluster)  [unwired: 15 in]
        n104 = call-dynamic "SetAD2_SDK.vi"("object in"=w256, "AD2_SDK"=w251) -> ("object out"=w255:refnum<class "Application.lvclass">)  [unwired: 16 in, 1 out]
        n105 = call-dynamic "FireUpdateStatus.vi"("object in"=w255, "Status"="MSO Configured") -> ("object out"=w249:refnum<class "Application.lvclass">)  [unwired: 16 in, 1 out]
      }
      frame "AD2MSORead" {
        n106 = call-dynamic "GetAD2_SDK.vi"("object in"=w267) -> ("object out"=w266:refnum<class "Application.lvclass">, "AD2_SDK"=w264:refnum<class "AD2_SDK.lvclass">)  [unwired: 16 in, 1 out]
        n107 = call-dynamic "ReadMSO.vi"("object in"=w264, "error in (no error)"=w262) -> ("object out"=w263:refnum<class "AD2_SDK.lvclass">, "Channels array"=→"Waveform Graph":waveform(dbl)[], "error out"=w261:errorcluster)  [unwired: 15 in]
        n108 = call-dynamic "SetAD2_SDK.vi"("object in"=w266, "AD2_SDK"=w263) -> ("object out"=w265:refnum<class "Application.lvclass">)  [unwired: 16 in, 1 out]
        n109 = call-dynamic "FireUpdateStatus.vi"("object in"=w265, "Status"="MSO Read") -> ("object out"=w260:refnum<class "Application.lvclass">)  [unwired: 16 in, 1 out]
      }
      frame "AD2Trigg" {
        n110 = call-dynamic "GetAD2_SDK.vi"("object in"=w276, "error in (no error)"=w272) -> ("object out"=w275:refnum<class "Application.lvclass">, "AD2_SDK"=w271:refnum<class "AD2_SDK.lvclass">, "error out"=w269:errorcluster)  [unwired: 15 in]
        n111 = call-dynamic "PCTrig.vi"("object in"=w271, "error in (no error)"=w269) -> ("object out"=w270:refnum<class "AD2_SDK.lvclass">, "error out"=w268:errorcluster)  [unwired: 16 in]
        n112 = call-dynamic "SetAD2_SDK.vi"("object in"=w275, "AD2_SDK"=w270, "error in (no error)"=w268) -> ("object out"=w274:refnum<class "Application.lvclass">, "error out"=w273:errorcluster)  [unwired: 15 in]
      }
      frame "PeltierInit" {
        n113 = call-dynamic "GetTC0608.vi"("object in"=w283) -> ("object out"=w285:refnum<class "Application.lvclass">, "TC0608"=w287:refnum<class "TC0608.lvclass">)  [unwired: 16 in, 1 out]
        n114 = call "TC0608_Init.vi"("object in"=w287, "VISA resource name"="Peltier VISA resource name", "error in (no error)"=w280) -> ("object out"=w286:refnum<class "TC0608.lvclass">, "error out"=w281:errorcluster)  [unwired: 15 in]
        n115 = call-dynamic "SetTC0608.vi"("object in"=w285, "TC0608"=w286) -> ("object out"=w284:refnum<class "Application.lvclass">)  [unwired: 16 in, 1 out]
        n116 = call-dynamic "UpdateStatus.vi"("object in"=w284, "Status"="Peltier Initialized") -> ("object out"=w279:refnum<class "Application.lvclass">)  [unwired: 16 in, 1 out]
        "Peltier is On" <- TRUE ("Peltier is On")
      }
      frame "PeltierRead" {
        n117 = call-dynamic "GetTC0608.vi"("object in"=w293) -> ("object out"=w295:refnum<class "Application.lvclass">, "TC0608"=w292:refnum<class "TC0608.lvclass">)  [unwired: 16 in, 1 out]
        n118 = call-dynamic "ReadTemperature.vi"("object in"=w292, "error in (no error)"=w290) -> ("object out"=w291:refnum<class "TC0608.lvclass">, "temperature (C)"=→"Temperature (C)":dbl, "error out"=w289:errorcluster)  [unwired: 15 in]
        n119 = call-dynamic "SetTC0608.vi"("object in"=w295, "TC0608"=w291) -> ("object out"=w294:refnum<class "Application.lvclass">)  [unwired: 16 in, 1 out]
      }
      frame "CetoniCheckLevelAndRefill" {
        n120 = call-dynamic "GetCetoniPump.vi"("object in"=w310, "error in (no error)"=w307) -> ("object out"=w296:refnum<class "Application.lvclass">, "CetoniPump"=w306:refnum<class "CetoniPump.lvclass">, "error out"=w298:errorcluster)  [unwired: 15 in]
        n121 = call-dynamic "ReadStatus.vi"("object in"=w306, "index"="index", "error in (no error)"=w298) -> ("object out"=w304:refnum<class "CetoniPump.lvclass">, "Fill Level"=w301:dbl, "error out"=w303:errorcluster)  [unwired: 12 in, 2 out]
        n122 = Less Or Equal?(x=w301, y="refill below level") -> (x <= y?=w302:bool)
        n123 = case shown="True" w302 {
          tunnel: "index" -> [_ w323]
          tunnel: w304 -> [w312 w319]
          tunnel: w303 -> [w311 w321]
          tunnel: [w312 w316] -> w299
          tunnel: [w311 w313] -> w297
          tunnel: w296 -> [_ w318]
          tunnel: w296 -> [_ w315]
          frame False {
          }
          frame True {
            n124 = call-dynamic "FireUpdateStatus.vi"("object in"=w318, "Status"="refilling") -> ()  [unwired: 16 in, 2 out]
            n125 = call-dynamic "Refill.vi"("object in"=w319, "index"=w323, "error in (no error)"=w321) -> ("object out"=w324:refnum<class "CetoniPump.lvclass">, "error out"=w322:errorcluster)  [unwired: 15 in]
            n126 = while {
              tunnel: w323 -> [w335]
              shift-right: [w325] -> w316
              shift-left: w324 -> [w336]
              shift-right: [w333] -> w313
              shift-left: w322 -> [w334]
              shift-right: [FALSE] -> _
              shift-left: TRUE -> [w327]
              stop <- w328 stop-if-true
              n127 = call-dynamic "ReadStatus.vi"("object in"=w336, "index"=w335, "error in (no error)"=w334) -> ("object out"=w325:refnum<class "CetoniPump.lvclass">, "Is pumping"=w331:bool, "error out"=w333:errorcluster)  [unwired: 12 in, 2 out]
              n128 = call "Elapsed Time"("Time Target (s)"="Timeout Refill", "Reset"=w327) -> ("Time has Elapsed"=w329:bool)  [unwired: 10 in, 7 out]
              n129 = Not(x=w331) -> (.not. x?=w330:bool)
              n130 = Or(x=w330, y=w329) -> (x .or. y?=w328:bool)
            }
            n131 = call-dynamic "FireUpdateStatus.vi"("object in"=w315, "Status"="refill complete", "error in (no error)"=w313) -> ()  [unwired: 15 in, 2 out]
          }
        }
        n132 = call-dynamic "SetCetoniPump.vi"("object in"=w296, "CetoniPump"=w299, "error in (no error)"=w297) -> ("object out"=w309:refnum<class "Application.lvclass">, "error out"=w308:errorcluster)  [unwired: 15 in]
      }
      frame "CetoniConfigureSyringe" {
        n133 = call-dynamic "GetCetoniPump.vi"("object in"=w347, "error in (no error)"=w343) -> ("object out"=w344:refnum<class "Application.lvclass">, "CetoniPump"=w342:refnum<class "CetoniPump.lvclass">, "error out"=w338:errorcluster)  [unwired: 15 in]
        n134 = call-dynamic "ConfigureSyringe.vi"("object in"=w342, "index"="index configure syringe", "SyringeSettings"="SyringeSettings", "error in (no error)"=w338) -> ("object out"=w341:refnum<class "CetoniPump.lvclass">, "error out"=w337:errorcluster)  [unwired: 14 in]
        n135 = call-dynamic "SetCetoniPump.vi"("object in"=w344, "CetoniPump"=w341, "error in (no error)"=w337) -> ("object out"=w346:refnum<class "Application.lvclass">, "error out"=w345:errorcluster)  [unwired: 15 in]
      }
      frame "CetoniEmpty" {
        n136 = Variant To Data(error in=w353, Variant=w355) -> (data=w348:i32, error out=w354:errorcluster)  [unwired: 1 in]
        n137 = call-dynamic "GetCetoniPump.vi"("object in"=w359, "error in (no error)"=w354) -> ("object out"=w356:refnum<class "Application.lvclass">, "CetoniPump"=w352:refnum<class "CetoniPump.lvclass">, "error out"=w350:errorcluster)  [unwired: 15 in]
        n138 = call-dynamic "Empty.vi"("object in"=w352, "index"=w348, "error in (no error)"=w350) -> ("object out"=w351:refnum<class "CetoniPump.lvclass">, "error out"=w349:errorcluster)  [unwired: 15 in]
        n139 = call-dynamic "SetCetoniPump.vi"("object in"=w356, "CetoniPump"=w351, "error in (no error)"=w349) -> ("object out"=w358:refnum<class "Application.lvclass">, "error out"=w357:errorcluster)  [unwired: 15 in]
      }
      frame "CetoniGoToLevel" {
        # "Updates Control with coerced\nvalues"
        n140 = local read "GoToLevelSettings"() -> (w363:T4)
        n141 = Variant To Data(error in=w364, type=w363, Variant=w366) -> (data=w362:T4, error out=w365:errorcluster)
        n142 = call-dynamic "GetCetoniPump.vi"("object in"=w375, "error in (no error)"=w365) -> ("object out"=w372:refnum<class "Application.lvclass">, "CetoniPump"=w369:refnum<class "CetoniPump.lvclass">, "error out"=w371:errorcluster)  [unwired: 15 in]
        n143 = call-dynamic "SetFillLevel.vi"("object in"=w369, "GoToLevelSettings"=w362, "error in (no error)"=w371) -> ("object out"=w368:refnum<class "CetoniPump.lvclass">, "Coerced Level"=w367:dbl, "Coerced Flow"=w361:dbl, "error out"=w370:errorcluster)  [unwired: 12 in, 1 out]
        n144 = Bundle By Name(cluster=w362, "Level(ml)"=w367, "Flow"=w361) -> (w360:T4)
        n145 = call-dynamic "SetCetoniPump.vi"("object in"=w372, "CetoniPump"=w368, "error in (no error)"=w370) -> ("object out"=w374:refnum<class "Application.lvclass">, "error out"=w373:errorcluster)  [unwired: 15 in]
        n146 = local write "GoToLevelSettings"(w360) -> ()
      }
      frame "CetoniInit" {
        n147 = call-dynamic "GetCetoniPump.vi"("object in"=w388, "error in (no error)"=w387) -> ("object out"=w385:refnum<class "Application.lvclass">, "CetoniPump"=w384:refnum<class "CetoniPump.lvclass">, "error out"=w382:errorcluster)  [unwired: 15 in]
        n148 = call "CetoniPump_Init.vi"("object in"=w384, "Device Configuration Path"="Device Configuration Folder", "error in (no error)"=w382) -> ("object out"=w383:refnum<class "CetoniPump.lvclass">, "error out"=w381:errorcluster)  [unwired: 15 in]
        n149 = call-dynamic "SetCetoniPump.vi"("object in"=w385, "CetoniPump"=w383, "error in (no error)"=w381) -> ("object out"=w378:refnum<class "Application.lvclass">, "error out"=w386:errorcluster)  [unwired: 15 in]
        n150 = call-dynamic "FireUpdateStatus.vi"("object in"=w378, "Status"="Syringe Pump Initialized") -> ("object out"=w377:refnum<class "Application.lvclass">)  [unwired: 16 in, 1 out]
        "Pump is On" <- TRUE ("Pump is On")
      }
      frame "CetoniReadStatus" {
        n151 = call-dynamic "GetCetoniPump.vi"("object in"=w401, "error in (no error)"=w398) -> ("object out"=w399:refnum<class "Application.lvclass">, "CetoniPump"=w397:refnum<class "CetoniPump.lvclass">, "error out"=w395:errorcluster)  [unwired: 15 in]
        n152 = call-dynamic "ReadStatusAllPumps.vi"("object in"=w397, "error in (no error)"=w395) -> ("object out"=w396:refnum<class "CetoniPump.lvclass">, "Array"=→"Pump Status":T1, "error out"=w394:errorcluster)  [unwired: 15 in]
        n153 = call-dynamic "SetCetoniPump.vi"("object in"=w399, "CetoniPump"=w396, "error in (no error)"=w394) -> ("object out"=w391:refnum<class "Application.lvclass">, "error out"=w400:errorcluster)  [unwired: 15 in]
        n154 = local read "Pump: Read Status"() -> (w389:bool)
        n155 = case shown="True" w389 {
          tunnel: "CetoniReadStatus" ("Message") -> [_ w405]
          tunnel: w391 -> [w402 w404]
          tunnel: [w402 w403] -> w390
          frame False {
          }
          frame True {
            n156 = call-dynamic "EnqueueMain.vi"("object in"=w404, "Message"=w405) -> ("object out"=w403:refnum<class "Application.lvclass">)  [unwired: 16 in, 1 out]
          }
        }
      }
      frame "CetoniReferenceMove" {
        n157 = call-dynamic "GetCetoniPump.vi"("object in"=w416, "error in (no error)"=w412) -> ("object out"=w413:refnum<class "Application.lvclass">, "CetoniPump"=w411:refnum<class "CetoniPump.lvclass">, "error out"=w408:errorcluster)  [unwired: 15 in]
        n158 = call-dynamic "GetConnectedPumps.vi"("object in"=w411) -> ("object out"=w410:refnum<class "CetoniPump.lvclass">, "ConnectedPumps"=w406:T20)  [unwired: 16 in, 1 out]
        n159 = for {
          shift-right: [w420] -> w409
          shift-left: w410 -> [w421]
          shift-right: [w418] -> w407
          shift-left: w408 -> [w419]
          tunnel: w406 -> [_] mode=indexing
          i -> [w417]
          n160 = call-dynamic "ReferenceMove.vi"("object in"=w421, "index"=w417, "error in (no error)"=w419) -> ("object out"=w420:refnum<class "CetoniPump.lvclass">, "error out"=w418:errorcluster)  [unwired: 15 in]
        }
        n161 = call-dynamic "SetCetoniPump.vi"("object in"=w413, "CetoniPump"=w409, "error in (no error)"=w407) -> ("object out"=w415:refnum<class "Application.lvclass">, "error out"=w414:errorcluster)  [unwired: 15 in]
      }
      frame "CetoniRefill" {
        n162 = Variant To Data(error in=w427, Variant=w429) -> (data=w422:i32, error out=w428:errorcluster)  [unwired: 1 in]
        n163 = call-dynamic "GetCetoniPump.vi"("object in"=w433, "error in (no error)"=w428) -> ("object out"=w430:refnum<class "Application.lvclass">, "CetoniPump"=w426:refnum<class "CetoniPump.lvclass">, "error out"=w424:errorcluster)  [unwired: 15 in]
        n164 = call-dynamic "Refill.vi"("object in"=w426, "index"=w422, "error in (no error)"=w424) -> ("object out"=w425:refnum<class "CetoniPump.lvclass">, "error out"=w423:errorcluster)  [unwired: 15 in]
        n165 = call-dynamic "SetCetoniPump.vi"("object in"=w430, "CetoniPump"=w425, "error in (no error)"=w423) -> ("object out"=w432:refnum<class "Application.lvclass">, "error out"=w431:errorcluster)  [unwired: 15 in]
      }
      frame "CetoniStopPumps" {
        n166 = call-dynamic "GetCetoniPump.vi"("object in"=w442, "error in (no error)"=w438) -> ("object out"=w439:refnum<class "Application.lvclass">, "CetoniPump"=w437:refnum<class "CetoniPump.lvclass">, "error out"=w435:errorcluster)  [unwired: 15 in]
        n167 = call-dynamic "StopAllPumps.vi"("object in"=w437, "error in (no error)"=w435) -> ("object out"=w436:refnum<class "CetoniPump.lvclass">, "error out"=w434:errorcluster)  [unwired: 16 in]
        n168 = call-dynamic "SetCetoniPump.vi"("object in"=w439, "CetoniPump"=w436, "error in (no error)"=w434) -> ("object out"=w441:refnum<class "Application.lvclass">, "error out"=w440:errorcluster)  [unwired: 15 in]
      }
      frame "ChangeFrequency" {
        n169 = Variant To Data(error in=w449, Variant=w451) -> (data=w446:dbl, error out=w450:errorcluster)  [unwired: 1 in]
        n170 = call-dynamic "GetAFG3022B.vi"("object in"=w452) -> ("object out"=w455:refnum<class "Application.lvclass">, "AFG3022B"=w454:refnum<class "AFG3022B.lvclass">)  [unwired: 16 in, 1 out]
        n171 = call-dynamic "Frequency Change Channel 1.vi"("object in"=w454, "Frequency (1000 Hz)"=w446) -> ("object out"=w453:refnum<class "AFG3022B.lvclass">)  [unwired: 16 in, 1 out]
        n172 = Number To Fractional String(number=w446) -> (F-format string=w444:string)  [unwired: 3 in]
        n173 = Concatenate Strings("Changed Frequency: " ("Status"), w444) -> (w445:string)
        n174 = call-dynamic "SetAFG3022B.vi"("object in"=w455, "AFG3022B"=w453) -> ("object out"=w448:refnum<class "Application.lvclass">)  [unwired: 16 in, 1 out]
        n175 = call-dynamic "FireUpdateStatus.vi"("object in"=w448, "Status"=w445) -> ("object out"=w447:refnum<class "Application.lvclass">)  [unwired: 16 in, 1 out]
      }
      frame "ChangeVoltage" {
        n176 = Variant To Data(error in=w465, Variant=w467) -> (data=w457:dbl, error out=w466:errorcluster)  [unwired: 1 in]
        n177 = call-dynamic "GetAFG3022B.vi"("object in"=w468) -> ("object out"=w469:refnum<class "Application.lvclass">, "AFG3022B"=w458:refnum<class "AFG3022B.lvclass">)  [unwired: 16 in, 1 out]
        n178 = Wait (ms)(milliseconds to wait=u32 500) -> ()  [unwired: 1 out]
        n179 = call-dynamic "Change Voltage Channel 1.vi"("object in"=w458, "Amplitude (1 Vpp)"=w457) -> ("object out"=w459:refnum<class "AFG3022B.lvclass">)  [unwired: 16 in, 1 out]
        n180 = Number To Fractional String(number=w457) -> (F-format string=w461:string)  [unwired: 3 in]
        n181 = Concatenate Strings("Changed Voltage: " ("Status"), w461) -> (w462:string)
        n182 = call-dynamic "SetAFG3022B.vi"("object in"=w469, "AFG3022B"=w459) -> ("object out"=w464:refnum<class "Application.lvclass">)  [unwired: 16 in, 1 out]
        n183 = call-dynamic "FireUpdateStatus.vi"("object in"=w464, "Status"=w462) -> ("object out"=w463:refnum<class "Application.lvclass">)  [unwired: 16 in, 1 out]
      }
      frame "Error" {
        # "#CodeRecommended - If you ever change the name of this \"Error\" message, you'll need to update the name in the Check Loop Error.vi as well."
        # "#CodeRecommended - Consider creating a system for logging errors in some way. These errors are for notification purposes only. Handling of specific errors should be performed in the message frames that generated the error."
        # "Error - Display an error dialog. This message is sent by the \"Error Handler\" VIs at the end of other loops in this application."
        n184 = Variant To Data(error in=w476, type=errorcluster {"status"=FALSE, "code"=0, "source"=""} ("error constant"), Variant=w475) -> (data=w473:errorcluster, error out=w472:errorcluster)
        n185 = call <vilib>:"Simple Error Handler.vi"("error in (no error)"=w473) -> ()  [unwired: 4 in, 5 out]
        n186 = Merge Errors(w472) -> (w471:errorcluster)
      }
      frame "Exit" {
        # "Stop the VI"
        # "Release the message queue reference"
        # "#CodeNeeded - Add any required cleanup code here. Note that if 'Exit' was called as a result of an error, an error dialog will be displayed. Add any custom error handling for an 'Exit' condition here as well."
        # "Exit - Exit the application."
        n187 = call <vilib>:"Simple Error Handler.vi"("error in (no error)"=w478) -> ("error out"=w477:errorcluster)  [unwired: 4 in, 4 out]
        n188 = call-dynamic "FireStopEvent.vi"("object in"=w480, "error in (no error)"=w477) -> ("object out"=w481:refnum<class "Application.lvclass">, "error out"=w479:errorcluster)  [unwired: 16 in]
      }
      frame "FuncInit" {
        n189 = call-dynamic "GetAFG3022B.vi"("object in"=w492) -> ("object out"=w493:refnum<class "Application.lvclass">, "AFG3022B"=w491:refnum<class "AFG3022B.lvclass">)  [unwired: 16 in, 1 out]
        n190 = call "AFG3022B_Init.vi"("object in"=w491, "VISA resource name"="Function Generator", "error in (no error)"=w487) -> ("object out"=w490:refnum<class "AFG3022B.lvclass">, "error out"=w488:errorcluster)  [unwired: 15 in]
        n191 = call-dynamic "SetAFG3022B.vi"("object in"=w493, "AFG3022B"=w490) -> ("object out"=w485:refnum<class "Application.lvclass">)  [unwired: 16 in, 1 out]
        n192 = call-dynamic "FireUpdateStatus.vi"("object in"=w485, "Status"="Function Generator Initialized") -> ("object out"=w484:refnum<class "Application.lvclass">)  [unwired: 16 in, 1 out]
        "Func is On" <- TRUE ("Func is On")
      }
      frame "Initialize" {
        # "Initialize - All initialization work should take place in this message, since other loops can potentially enqueue messages that execute immediately after this one."
        n193 = Build Array("CoriolisInit", "CetoniInit", "HamamatsuInit", "AD2Init", "OscilloscopeInit" ("element"), "PeltierInit" ("element")) -> (w501:string[])
        n194 = for {
          shift-right: [w505] -> w499
          shift-left: w498 -> [w506]
          tunnel: w501 -> [w504] mode=indexing
          n195 = call-dynamic "EnqueueMain.vi"("object in"=w506, "Message"=w504) -> ("object out"=w505:refnum<class "Application.lvclass">)  [unwired: 16 in, 1 out]
        }
      }
      frame "OscilloscopeInit" {
        n196 = call-dynamic "GetTBS2000.vi"("object in"=w513) -> ("object out"=w512:refnum<class "Application.lvclass">, "TBS2000Series"=w514:refnum<class "TBS2000Series.lvclass">)  [unwired: 16 in, 1 out]
        n197 = call "TBS2000Series_Init.vi"("object in"=w514, "VISA resource name"="Oscilloscope", "error in (no error)"=w516) -> ("object out"=w511:refnum<class "TBS2000Series.lvclass">, "error out"=w515:errorcluster)  [unwired: 15 in]
        n198 = call-dynamic "Set TBS2000.vi"("object in"=w512, "TBS2000Series"=w511) -> ("object out"=w510:refnum<class "Application.lvclass">)  [unwired: 16 in, 1 out]
        n199 = call-dynamic "FireUpdateStatus.vi"("object in"=w510, "Status"="Oscilloscope Initialized") -> ("object out"=w509:refnum<class "Application.lvclass">)  [unwired: 16 in, 1 out]
        "Oscilloscope is On" <- TRUE ("Oscilloscope is On")
      }
      frame "MeasurePowerOsc" {
        n200 = call-dynamic "GetTBS2000.vi"("object in"=w526) -> ("object out"=w525:refnum<class "Application.lvclass">, "TBS2000Series"=w523:refnum<class "TBS2000Series.lvclass">)  [unwired: 16 in, 1 out]
        n201 = call-dynamic "Read Osc. Energy Density.vi"("object in"=w523, "Oscilloscope"="Oscilloscope Test", "error in (no error)"=w519) -> ("object out"=w522:refnum<class "TBS2000Series.lvclass">, "Oscilloscope Results"=→"Oscilloscope Results Test":T6, "error out"=w520:errorcluster)  [unwired: 10 in]
        n202 = call-dynamic "Set TBS2000.vi"("object in"=w525, "TBS2000Series"=w522) -> ("object out"=w524:refnum<class "Application.lvclass">)  [unwired: 16 in, 1 out]
      }
      frame "ReadOscilloscopeChannel" {
        n203 = call-dynamic "GetTBS2000.vi"("object in"=w532) -> ("object out"=w531:refnum<class "Application.lvclass">, "TBS2000Series"=w530:refnum<class "TBS2000Series.lvclass">)  [unwired: 16 in, 1 out]
        n204 = call-dynamic "Read Piezo Prefocus.vi"("object in"=w530, "Source (1: Channel 1)"="Source (1: Channel 1)") -> ("object out"=w529:refnum<class "TBS2000Series.lvclass">, "Frequency"=→"Frequency":dbl, "Peak-to-Peak"=→"Peak-to-Peak":dbl)  [unwired: 13 in, 2 out]
        n205 = call-dynamic "Set TBS2000.vi"("object in"=w531, "TBS2000Series"=w529) -> ("object out"=w533:refnum<class "Application.lvclass">)  [unwired: 16 in, 1 out]
      }
      frame "FuncOscSave" {
        n206 = Variant To Data(error in=w551, type=T18 {"Voltages"=0.0, "Numeric"=0.0, "selected path"=path ""} ("output cluster"), Variant=w562) -> (data=w544:T18, error out=w552:errorcluster)
        n207 = call-dynamic "GetTC0608.vi"("object in"=w539) -> ("object out"=w541:refnum<class "Application.lvclass">, "TC0608"=w538:refnum<class "TC0608.lvclass">)  [unwired: 16 in, 1 out]
        n208 = call-dynamic "ReadTemperature.vi"("object in"=w538) -> ("object out"=w537:refnum<class "TC0608.lvclass">, "temperature (C)"=w536:dbl)  [unwired: 16 in, 1 out]
        "temperature (C)" <- w536
        n209 = call-dynamic "SetTC0608.vi"("object in"=w541, "TC0608"=w537) -> ("object out"=w540:refnum<class "Application.lvclass">)  [unwired: 16 in, 1 out]
        n210 = Unbundle(w544) -> ("Voltages"=→"Voltages":dbl, "Numeric"=→"Frequencies":dbl)  [unwired: 1 out]
        n211 = call-dynamic "GetTBS2000.vi"("object in"=w540) -> ("object out"=w561:refnum<class "Application.lvclass">, "TBS2000Series"=w560:refnum<class "TBS2000Series.lvclass">)  [unwired: 16 in, 1 out]
        n212 = call-dynamic "Read Piezo Prefocus.vi"("object in"=w560, "Source (1: Channel 1)"="Oscilloscope Source", "error in (no error)"=w552) -> ("object out"=w559:refnum<class "TBS2000Series.lvclass">, "Frequency"=w554:dbl, "Peak-to-Peak"=w553:dbl, "error out"=w548:errorcluster)  [unwired: 12 in, 1 out]
        "Frequency (Osc.)" <- w554
        "Voltage (Osc.)" <- w553
        n213 = call-dynamic "Set TBS2000.vi"("object in"=w561, "TBS2000Series"=w559) -> ("object out"=w556:refnum<class "Application.lvclass">)  [unwired: 16 in, 1 out]
        n214 = Bundle("Frequency"=w554, "Peak-to-Peak"=w553, "temperature (C)"=w536) -> (w549:T21)  [unwired: 1 in]
        n215 = call-dynamic "GetSaveData.vi"("object in"=w556) -> ("object out"=w557:refnum<class "Application.lvclass">, "SaveData"=w550:refnum<class "SaveData.lvclass">)  [unwired: 16 in, 1 out]
        n216 = call-dynamic "Exp_Test 1.vi"("object in"=w550, "output cluster"=w544, "Oscilloscope Results"=w549, "error in (no error)"=w548) -> ("object out"=w546:refnum<class "SaveData.lvclass">, "error out"=w547:errorcluster)  [unwired: 14 in]
        n217 = call-dynamic "SetSaveData.vi"("object in"=w557, "SaveData"=w546) -> ("object out"=w555:refnum<class "Application.lvclass">)  [unwired: 16 in, 1 out]
      }
      frame "SaveDataEacExperiment" {
        n218 = call-dynamic "GetTC0608.vi"("object in"=w583) -> ("object out"=w582:refnum<class "Application.lvclass">, "TC0608"=w581:refnum<class "TC0608.lvclass">)  [unwired: 16 in, 1 out]
        n219 = call-dynamic "ReadTemperature.vi"("object in"=w581, "error in (no error)"=w579) -> ("object out"=w580:refnum<class "TC0608.lvclass">, "temperature (C)"=w567:dbl, "error out"=w569:errorcluster)  [unwired: 15 in]
        "Temperatur (C)" <- w567
        n220 = call-dynamic "SetTC0608.vi"("object in"=w582, "TC0608"=w580) -> ("object out"=w577:refnum<class "Application.lvclass">)  [unwired: 16 in, 1 out]
        n221 = call-dynamic "GetTBS2000.vi"("object in"=w577) -> ("object out"=w578:refnum<class "Application.lvclass">, "TBS2000Series"=w576:refnum<class "TBS2000Series.lvclass">)  [unwired: 16 in, 1 out]
        n222 = Variant To Data(Variant=w566) -> (data=w565:T8)  [unwired: 2 in, 1 out]
        n223 = call-dynamic "Read Osc. Energy Density.vi"("object in"=w576, "error in (no error)"=w569) -> ("object out"=w575:refnum<class "TBS2000Series.lvclass">, "error out"=w570:errorcluster)  [unwired: 11 in, 1 out]
        n224 = call-dynamic "Set TBS2000.vi"("object in"=w578, "TBS2000Series"=w575) -> ("object out"=w563:refnum<class "Application.lvclass">)  [unwired: 16 in, 1 out]
        n225 = call-dynamic "GetSaveData.vi"("object in"=w563) -> ("object out"=w574:refnum<class "Application.lvclass">, "SaveData"=w573:refnum<class "SaveData.lvclass">)  [unwired: 16 in, 1 out]
        n226 = call "EacExperiment.vi"("object in"=w573, "Path"="SaveFolder", "Temperature (C)"=w567, "Experiment Settings"=w565, "error in (no error)"=w570) -> ("object out"=w572:refnum<class "SaveData.lvclass">, "error out"=w568:errorcluster)  [unwired: 13 in]
        n227 = call-dynamic "SetSaveData.vi"("object in"=w574, "SaveData"=w572) -> ("object out"=w571:refnum<class "Application.lvclass">)  [unwired: 16 in, 1 out]
      }
      frame "TakeNImages" {
        # "This Constants is set to give a 1ms pulse over 5ms span, pc triggered, and then wait for new trigger\nDo not Change unless you know how to set the DOs of the AD2"
        n228 = Variant To Data(error in=w587, type=T19 {"Minimum Time between frames"=10.0, "Number of Frames"=0} ("Image  Aquisition"), Variant=w590) -> (data=w586:T19, error out=w588:errorcluster)
        n229 = Unbundle By Name(w586) -> ("Minimum Time between frames"=w585:dbl, "Number of Frames"=w584:i32)
        n230 = call-dynamic "GetAD2_SDK.vi"("object in"=w594) -> ("object out"=w593:refnum<class "Application.lvclass">, "AD2_SDK"=w599:refnum<class "AD2_SDK.lvclass">, "error out"=w598:errorcluster)  [unwired: 16 in]
        n231 = call-dynamic "ConfigDO.vi"("object in"=w599, 2:T14 {"DO Trigger"={"secRun(0=Cont)"=0.005, "secWait"=0.0, "cRepeat(0=inf)"=0, "Repeat Trigger"=TRUE, "TrigrSrc"=enum."trigsrcPC"}, "CustomData"=[{"Data"=[FALSE, TRUE, FALSE, FALSE, FALSE, FALSE, FALSE, FALSE, FALSE, FALSE, FALSE, FALSE, FALSE, FALSE, FALSE, FALSE, FALSE, FALSE, FALSE, FALSE, FALSE, FALSE], "Freq"=1000.0, "#Bits"=100, "Enable"=TRUE, "IdleState"=0}, {"Data"=[], "Freq"=0.0, "#Bits"=0, "Enable"=FALSE, "IdleState"=0}, {"Data"=[], "Freq"=0.0, "#Bits"=0, "Enable"=FALSE, "IdleState"=0}, {"Data"=[], "Freq"=0.0, "#Bits"=0, "Enable"=FALSE, "IdleState"=0}, {"Data"=[], "Freq"=0.0, "#Bits"=0, "Enable"=FALSE, "IdleState"=0}, {"Data"=[], "Freq"=0.0, "#Bits"=0, "Enable"=FALSE, "IdleState"=0}, {"Data"=[], "Freq"=0.0, "#Bits"=0, "Enable"=FALSE, "IdleState"=0}, {"Data"=[], "Freq"=0.0, "#Bits"=0, "Enable"=FALSE, "IdleState"=0}, {"Data"=[], "Freq"=0.0, "#Bits"=0, "Enable"=FALSE, "IdleState"=0}, {"Data"=[], "Freq"=0.0, "#Bits"=0, "Enable"=FALSE, "IdleState"=0}, {"Data"=[], "Freq"=0.0, "#Bits"=0, "Enable"=FALSE, "IdleState"=0}, {"Data"=[], "Freq"=0.0, "#Bits"=0, "Enable"=FALSE, "IdleState"=0}, {"Data"=[], "Freq"=0.0, "#Bits"=0, "Enable"=FALSE, "IdleState"=0}]}, "error in (no error)"=w598) -> ("object out"=w596:refnum<class "AD2_SDK.lvclass">, "error out"=w597:errorcluster)  [unwired: 15 in]
        n232 = for {
          N: w584 -> [_]
          shift-right: [w604] -> w600
          shift-left: w597 -> [w609]
          shift-right: [w610] -> w601
          shift-left: w596 -> [w608]
          shift-right: [w606] -> w592
          shift-left: w593 -> [w607]
          tunnel: w585 -> [w602]
          stop <- w603 stop-if-true
          n233 = call-dynamic "PCTrig.vi"("object in"=w608, "error in (no error)"=w609) -> ("object out"=w610:refnum<class "AD2_SDK.lvclass">, "error out"=w605:errorcluster)  [unwired: 16 in]
          n234 = call-dynamic "Wait.vi"("object in"=w607, "Time to wait"=w602, "error in (no error)"=w605) -> ("object out"=w606:refnum<class "Application.lvclass">, "aborted"=w603:bool, "error out"=w604:errorcluster)  [unwired: 14 in]
        }
        n235 = call-dynamic "SetAD2_SDK.vi"("object in"=w592, "AD2_SDK"=w601, "error in (no error)"=w600) -> ("object out"=w595:refnum<class "Application.lvclass">)  [unwired: 15 in, 1 out]
      }
      frame "Wait" {
        n236 = Variant To Data(error in=w619, Variant=w621) -> (data=w620:dbl, error out=w616:errorcluster)  [unwired: 1 in]
        n237 = call-dynamic "FireUpdateStatus.vi"("object in"=w617, "Status"="waiting.....") -> ("object out"=w614:refnum<class "Application.lvclass">)  [unwired: 16 in, 1 out]
        n238 = call-dynamic "Wait.vi"("object in"=w614, "Time to wait"=w620, "error in (no error)"=w616) -> ("object out"=w618:refnum<class "Application.lvclass">, "error out"=w615:errorcluster)  [unwired: 14 in, 1 out]
        n239 = call-dynamic "FireUpdateStatus.vi"("object in"=w618, "Status"="wait complete") -> ("object out"=w612:refnum<class "Application.lvclass">)  [unwired: 16 in, 1 out]
      }
      frame Default {
        # "'Default' case only runs if there is a message that isn't defined in any of the other cases.  Output a programming error."
        n240 = xnode "Error Ring"("parameter 0"=w623) -> ("error out"=w624:errorcluster)
      }
    }
    n241 = call-dynamic "ErrorHandlerMainLoop.vi"("object in"=w210, "error in (no error)"=w213) -> ("object out"=w211:refnum<class "Application.lvclass">, "error out"=w212:errorcluster)  [unwired: 16 in]
  }
  n242 = Merge Errors(w5, w6) -> (w4:errorcluster)
  n243 = call-dynamic "CleanUp.vi"("object in"=w7, "error in (no error)"=w4) -> ("error out"=→"error out":errorcluster)  [unwired: 16 in, 1 out]
